vi "tcp_monitor_json_update_int.vi"(9 "Input":i32, 10 "keyString":string, 11 "Json Input":string="{\"code\": 111, \"msg\": \"success\", \"data\": {\"camera_udp_port\": 10001, \"radar_udp_port\": 17000, \"radar_decode_head\": \"AAAA5555\", \"tcp_server_port\": 8888, \"mcu_enable\": 1, \"ntp_enable\": 1, \"radar_get_edition_enable\": 1, \"mcu_get_edition_enable\": 1, \"infer_enable\": 1, \"cpu_min_to_restart_infer\": 20, \"camera_remote_enable\": 1, \"video_save\": 3, \"pronounce_english\": 0, \"zipx_s_service_restart_time_s\": -1, \"http_file_port\": -1, \"max_file_num\": 1000, \"max_file_size\": 2000000000, \"pic_timeSpan_min\": 5, \"mp4_timeSpan_min\": 4, \"pika_rabbitmq_enable\": 0, \"pika_sftp_enable\": 0, \"radar_alarm_score\": 455, \"camera_alarm_score\": 20, \"joint_alarm_score\": 150, \"camera_radar_h_offset_rad\": -0.01, \"confidence_min\": 0.55, \"radarOffset\": 0.0, \"autoMendRadarOffset\": 0, \"autoCalibration\": 0, \"H\": 2.4}}") -> (1 "Value out":i32, 3 "Json Output":string)   [LabVIEW 2022 SP3]
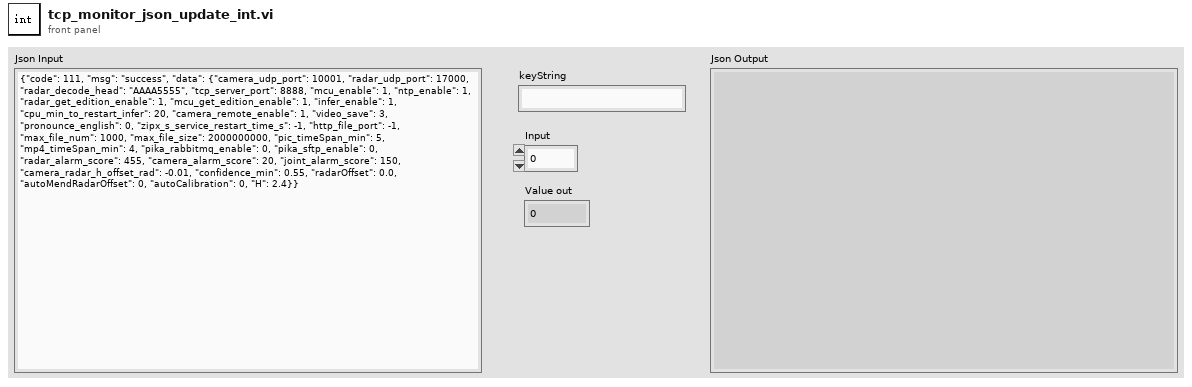
[diagram p1: front panel]
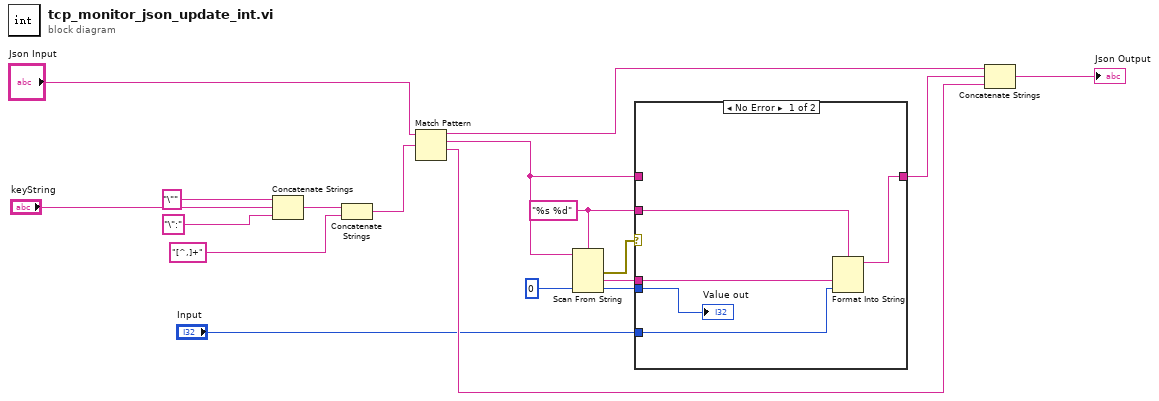
[diagram p0: block diagram]
diagram:
  w5 = "%s %d" ("format string")
  n1 = Concatenate Strings("\"" ("string"), "keyString", "\":" ("regular expression")) -> (w3:string)
  n2 = Concatenate Strings(w3, "[^,]+" ("string")) -> (w2:string)
  n3 = Match Pattern(string="Json Input", regular expression=w2) -> (before substring=w9:string, match substring=w10:string, after substring=w8:string)  [unwired: 1 in, 1 out]
  n4 = Scan From String(format string=w5, input string=w10, default 2=0) -> (error out=w11:errorcluster, output 1=w14:string, output 2=w16:i32)  [unwired: 3 in, 2 out]
  n5 = case shown="No Error" w11 {
    tunnel: w16 -> [w23 _]
    tunnel: w14 -> [w21 _]
    tunnel: w10 -> [_ w24]
    tunnel: [w19 w24] -> w7
    tunnel: w5 -> [w22 _]
    tunnel: "Input" -> [w20 _]
    frame No Error {
      n6 = Format Into String(format string=w22, w21, w20) -> (resulting string=w19:string)  [unwired: 2 in, 1 out]
      "Value out" <- w23
    }
    frame Error {
    }
  }
  n7 = Concatenate Strings(w9, w7, w8) -> (→"Json Output":string)
